vi "User.vi"   [LabVIEW 2019, in "xy_utilities.lvlib"]
uses:
  xy_utilities.lvlib
  User/User.lvclass
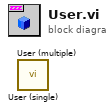
[diagram p0: block diagram]
diagram:
  n1 = call "User (single).vi"() -> ()  [unwired: 10 in, 2 out]
  n2 = call "User (multiple).vi"() -> ()  [unwired: 10 in, 2 out]
